vi "atividade 4.vi"(8 "error in (no error)":errorcluster, 9 "Filename":path=path "C:/Users/LSE/Documents/GitHub/Repo_Labview/ProjetoLabVIEW/Resources/Updated_EmulatedData_ThreePhase_FiveOutages.csv", 10 "Enable":bool=TRUE, 11 "Reset":bool) -> (0 "error out":errorcluster, 2 "Filename Out":path, 3 "Signals":dynamicdata(graph), 4 "EOF?":bool, 5 "Comment":string, 7 "Description":string)   [LabVIEW 2025]
doc: "<p><a href=\"nihelplauncher://docs/csh?context=lvcore_lvhowto_reading_using_expressvi\">Reads data from</a> a <a href=\"nihelplauncher://docs/csh?context=lvcore_lvhowto_labview_data_file\">text-based measurement file (<span class=\"Monospace\">.lvm</span>)</a> or <a href=\"nihelplauncher://docs/csh?context=lvcore_lvhowto_ni_test_data_exchange\">binary measurement file (<span class=\"Monospace\">.tdm</span> or <span class=\"Monospace\">.tdms</span>)</a>.</p>\n--------------------\n\nThis Express VI is configured as follows:\n\nFile Path:C:\\Users\\LSE\\Documents\\GitHub\\Repo_Labview\\ProjetoLabVIEW\\Resources\\Updated_EmulatedData_ThreePhase_FiveOutages.csv\nRead Generic Text Files:True\nFile Format: Text (LVM)\nDelimiter: Comma\nDecimal Point: . (dot)\nStart Row Data:2\nFirst Row is Channel: Names: True\nFirst Column is Time Channel: False\nTimestamp: Absolute\nAsk User To Choose File: True\nSegment Size: Retrieve segments of original size"
uses:
  <vilib>/express/express shared/ExFile.llb/ex_FileFormats.ctl
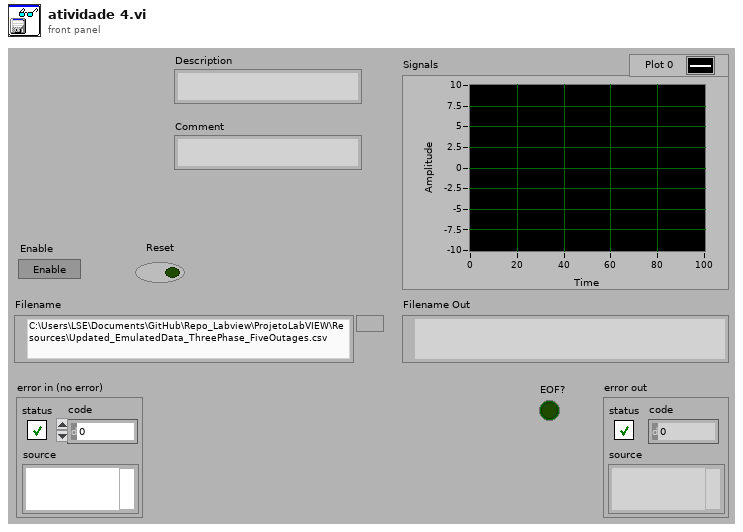
[diagram p1: front panel]
types:
  T1 = typedef "ex_FileFormats.ctl" = enum32{"lvm", "tdm", "tdms", "xlsx"}
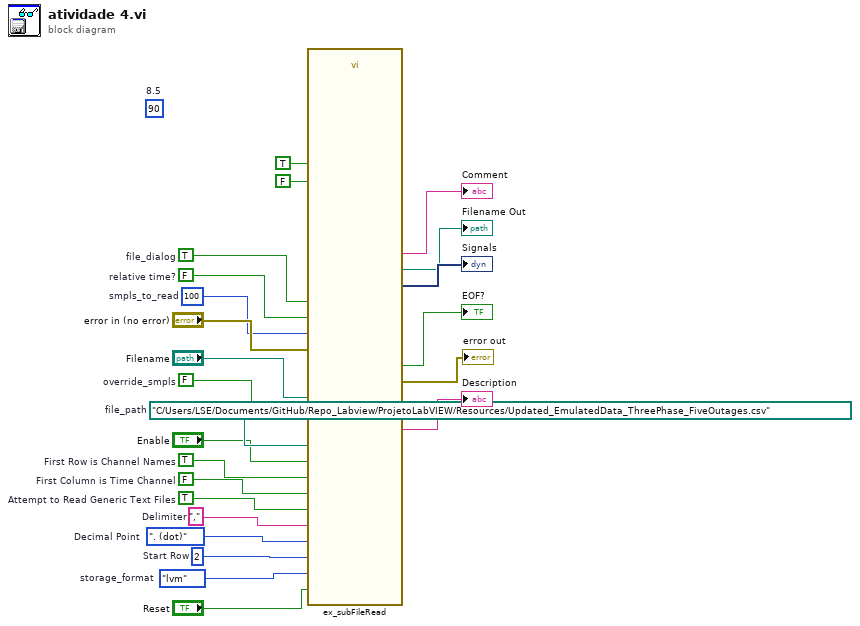
[diagram p0: block diagram]
diagram:
  (unwired) 90  # 8.5
  w6 = ","  # Delimiter
  w4 = ex_FileFormats."lvm"  # storage_format
  w7 = enum32{". (dot)", ", (comma)"}.". (dot)"  # Decimal Point
  w11 = 2  # Start Row
  w10 = TRUE  # Attempt to Read Generic Text Files
  w9 = FALSE  # First Column is Time Channel
  w8 = TRUE  # First Row is Channel Names
  w14 = path "C:/Users/LSE/Documents/GitHub/Repo_Labview/ProjetoLabVIEW/Resources/Updated_EmulatedData_ThreePhase_FiveOutages.csv"  # file_path
  w16 = FALSE  # relative time?
  w20 = FALSE  # override_smpls
  w21 = 100  # smpls_to_read
  w22 = TRUE  # file_dialog
  n1 = call <vilib>:"ex_subFileRead.vi"("file path in"="Filename", "First Column is Time Channel"=w9, "file dialog?"=w22, "relative time?"=w16, "Attempt to Read Generic Text Files"=w10, "samples to read"=w21, "error in (no error)"="error in (no error)", "delimiter"=w6, "First Row is Channel Names"=w8, "Decimal point"=w7, "static path in"=w14, "override samples"=w20, "Enable"="Enable", "Start Row"=w11, "storage_format"=w4, "single values"=FALSE, "Lock file"=TRUE, "Reset"="Reset") -> ("Description"=→"Description":string, "Comment"=→"Comment":string, "EOF?"=→"EOF?":bool, "file path out"=→"Filename Out":path, "Signals"=→"Signals":dynamicdata, "error out"=→"error out":errorcluster)  [unwired: 4 out]
